vi "19052 PreSet_SERIAL_NUMBER.vi"(1 "Serial number":string, 8 "error in (no error)":errorcluster, 11 "VISA resource in":refnum<visa-resource-name>) -> (0 "error out":errorcluster, 2 "output command":string, 3 "VISA resource out":refnum<visa-resource-name>)   [LabVIEW 2015]
uses:
  Type Definitions/serial__lot_part_number_states.ctl
panel:
  # "Set SERIAL number"
  # "Min 5 char, Max 13 char"
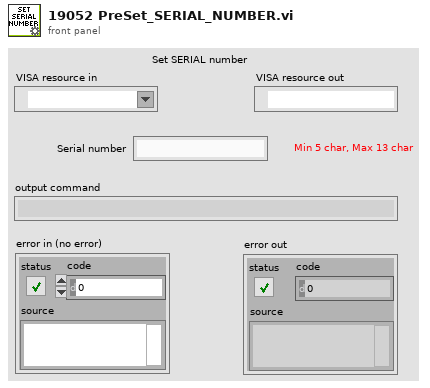
[diagram p1: front panel]
types:
  T1 = typedef "serial__lot_part_number_states.ctl" = enum16{"check <=UL", "check >=LL", "trim", "write", "Shutdown"}
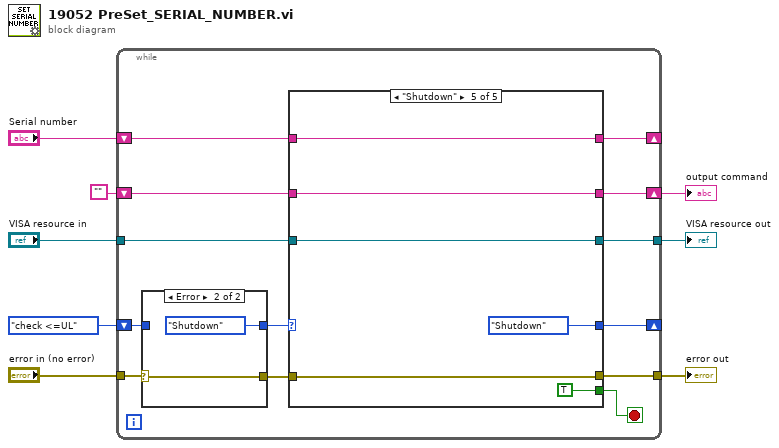
[diagram p0: block diagram]
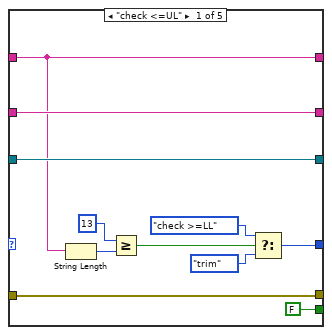
[diagram p3: hidden frame]
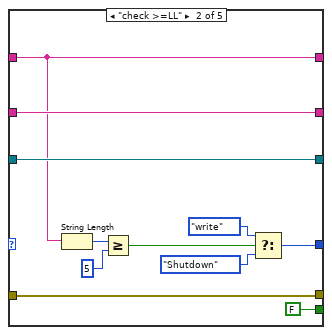
[diagram p4: hidden frame]
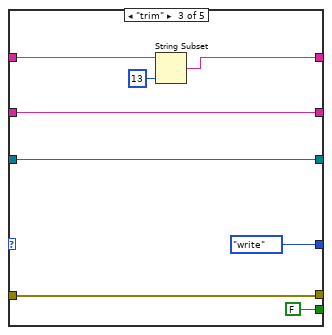
[diagram p5: hidden frame]
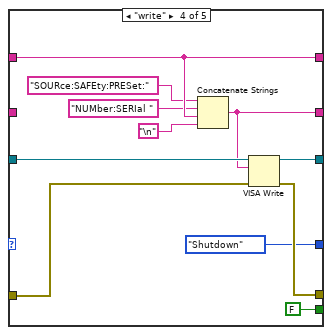
[diagram p6: hidden frame]
diagram:
  n1 = while {
    tunnel: "error in (no error)" -> [w20]
    shift-right: [w18] -> _
    shift-left: serial__lot_part_number_states."check <=UL" -> [w17]
    tunnel: "VISA resource in" -> [w16]
    tunnel: [w14] -> w5
    tunnel: [w13] -> w4
    shift-right: [w12] -> _
    shift-left: "Serial number" -> [w19]
    shift-right: [w11] -> w3
    shift-left: "" -> [w9]
    stop <- w10 stop-if-true
    n2 = case shown="Error" w20 {
      selector: w20 -> [w23 w24]
      tunnel: [w23 w24] -> w15
      tunnel: [w22 serial__lot_part_number_states."Shutdown"] -> w21
      tunnel: w17 -> [w22 _]
      frame No Error {
      }
      frame Error {
      }
    }
    n3 = case shown="\"Shutdown\"" w21 {
      tunnel: w19 -> [w28 w42 w53 w61 w70]
      tunnel: [w32 w41 serial__lot_part_number_states."write" serial__lot_part_number_states."Shutdown" serial__lot_part_number_states."Shutdown"] -> w18
      tunnel: w16 -> [w30 w46 w55 w65 w72]
      tunnel: w15 -> [w29 w45 w54 w64 w71]
      tunnel: [w29 w45 w54 w63 w71] -> w14
      tunnel: [w30 w46 w55 w62 w72] -> w13
      tunnel: [w28 w42 w51 w61 w70] -> w12
      tunnel: [w36 w47 w48 w59 w67] -> w11
      tunnel: [FALSE FALSE FALSE FALSE TRUE] -> w10
      tunnel: w9 -> [w36 w47 w48 _ w67]
      frame "check <=UL" {
        n4 = String Length(string=w28) -> (length=w34:i32)
        n5 = Greater Or Equal?(x=13 ("y"), y=w34) -> (x >= y?=w33:bool)
        n6 = Select(t=serial__lot_part_number_states."check >=LL", s=w33, f=serial__lot_part_number_states."trim") -> (s? t:f=w32:T1)
      }
      frame "check >=LL" {
        n7 = String Length(string=w42) -> (length=w44:i32)
        n8 = Greater Or Equal?(x=w44, y=5) -> (x >= y?=w39:bool)
        n9 = Select(t=serial__lot_part_number_states."write", s=w39, f=serial__lot_part_number_states."Shutdown") -> (s? t:f=w41:T1)
      }
      frame "trim" {
        n10 = String Subset(string=w53, length (rest)=13 ("length (rest)")) -> (substring=w51:string)  [unwired: 1 in]
      }
      frame "write" {
        n11 = Concatenate Strings("SOURce:SAFEty:PRESet:", "NUMber:SERIal ", w61, "\n") -> (w59:string)
        n12 = VISA Write(VISA resource name=w65, write buffer=w59, error in (no error)=w64) -> (VISA resource name out=w62:refnum<visa-resource-name>, error out=w63:errorcluster)  [unwired: 1 out]
      }
      frame "Shutdown" {
      }
    }
  }
  "error out" <- w5
  "VISA resource out" <- w4
  "output command" <- w3
